vi "read_file_type_extension_to_search.vi"(8 "error in (no error)":errorcluster, 11 "config_file_name":string) -> (0 "error out":errorcluster, 2 "extension_to_search":string, 3 "config_file_name_out":string)   [LabVIEW 2015]
uses:
  <vilib>/Utility/config.llb/Read Key (String).vi
  <vilib>/Utility/config.llb/NI_LVConfig.lvlib
panel:
  # "Devuelve datos de la sección FILE TYPE del archivo de configuración"
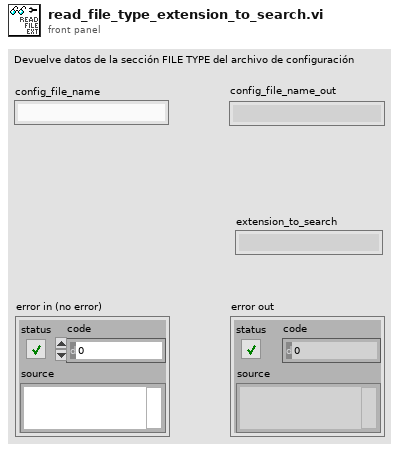
[diagram p1: front panel]
types:
  T1 = typedef "NI_LVConfig.lvlib/Config Data RefNum.ctl" = refnum<k1>
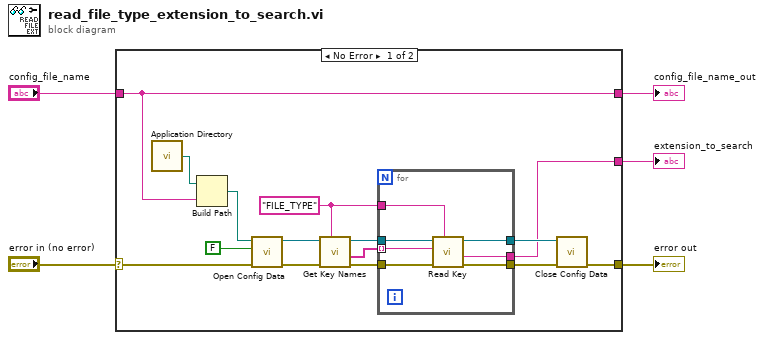
[diagram p0: block diagram]
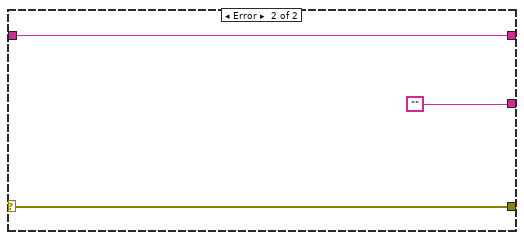
[diagram p2: hidden frame]
diagram:
  n1 = case shown="No Error" "error in (no error)" {
    selector: "error in (no error)" -> [w11 w30]
    tunnel: [w10 w30] -> w5
    tunnel: [w9 w29] -> w3
    tunnel: "config_file_name" -> [w9 w29]
    tunnel: [w6 ""] -> w1
    frame No Error {
      w16 = "FILE_TYPE" ("section")
      n2 = call <vilib>:"Application Directory.vi"() -> ("Application Directory"=w18:path)
      n3 = Build Path(base path=w18, name or relative path=w9) -> (appended path=w17:path)
      n4 = call <vilib>:"Open Config Data.vi"("error in (no error)"=w11, "create file if necessary (T)"=FALSE, "configuration file path"=w17) -> ("error out"=w20:errorcluster, "refnum"=w19:T1)  [unwired: 6 in, 1 out]
      n5 = call <vilib>:"Get Key Names.vi"("section"=w16, "error in (no error)"=w20, "refnum"=w19) -> ("error out"=w14:errorcluster, "key names"=w8:string[], "refnum out"=w15:T1)  [unwired: 5 in, 1 out]
      n6 = for {
        tunnel: w8 -> [w27] mode=indexing
        tunnel: [w26] -> w6
        tunnel: w16 -> [w25]
        tunnel: w15 -> [w24]
        tunnel: w14 -> [w23]
        tunnel: [w22] -> w13
        tunnel: [w21] -> w12
        n7 = call-poly <vilib>:"Read Key.vi"("section"=w25, "error in (no error)"=w23, "key"=w27, "refnum"=w24) -> ("error out"=w21:errorcluster, "value"=w26:string, "refnum out"=w22:T1)  [unwired: 4 in, 1 out]
      }
      n8 = call <vilib>:"Close Config Data.vi"("error in (no error)"=w12, "refnum"=w13) -> ("error out"=w10:errorcluster)  [unwired: 8 in, 1 out]
    }
    frame Error {
    }
  }
  "error out" <- w5
  "config_file_name_out" <- w3
  "extension_to_search" <- w1
